vi "Rx Message to Transfer Handle - RT.vi"(8 "error in":errorcluster, 9 "message":T2={"name"="", "message type"="BC to RT", "endpoint Tx"={"terminal address"=0, "subaddress"=0}, "endpoint Rx"={"terminal address"=0, "subaddress"=0}, "create timestamp channel"=FALSE, "mode code"=0, "number of words"=0, "parameters"=[]}, 11 "remote terminal handles":u64[](array[numeric])) -> (0 "error out":errorcluster, 2 "valid?":bool, 3 "Rx read info":T1)   [LabVIEW 2020, in "AIM MIL-STD-1553 Engine.lvlib" / "Implementation.lvlib" / "Rx Execution Unit.lvclass"]
uses:
  Rx Execution Unit.lvclass
  <instrlib>/BTI1553Lib/BTI1553LV.lvlib
  <instrlib>/BTI1553Lib/Public/Controls/1553 RT Transfer Type.ctl
  <instrlib>/BTI1553Lib/Public/Controls/1553 Transfer Direction.ctl
  Shared/Rx Read Info.ctl
  <instrlib>/BTI1553Lib/Private/RT/Configure/Get RT Xfer Handle.vi
  Shared/Address.ctl
  Shared/Terminal Endpoint.ctl
  Shared/Parameter Definition.ctl
  Shared/Message Type.ctl
  Shared/Message Definition.ctl
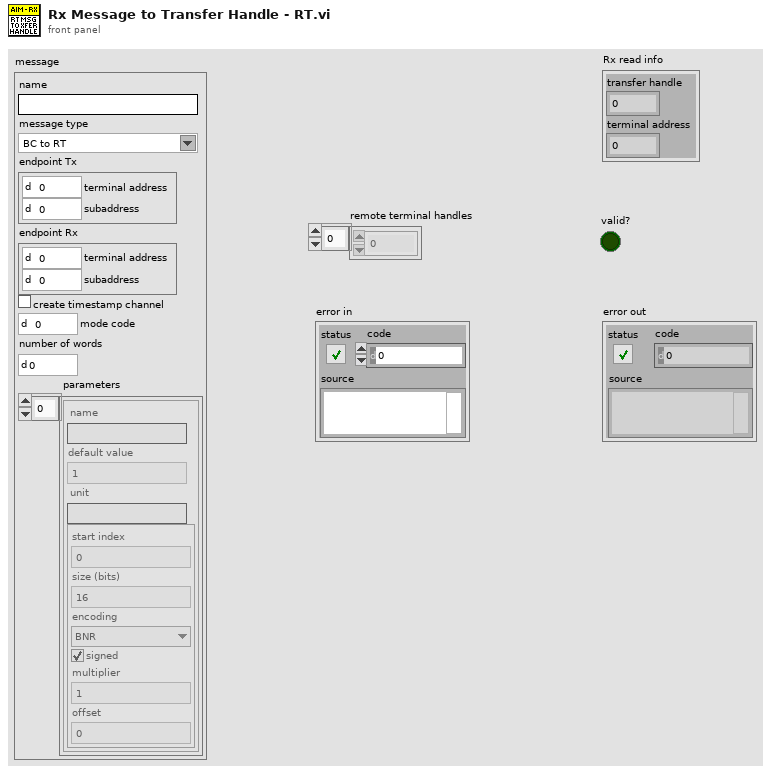
[diagram p1: front panel]
types:
  T1 = typedef "Rx Read Info.ctl" = cluster{"transfer handle":u64, "terminal address":u16}
  T2 = typedef "Message Definition.ctl" = cluster{"name":string, "message type":T3, "endpoint Tx":T4, "endpoint Rx":T4, "create timestamp channel":bool, "mode code":u16, "number of words":u16, "parameters":cluster{"name":string, "default value":dbl, "unit":string, "parameter definition":T6}[]}
  T3 = typedef "Message Type.ctl" = string
  T4 = typedef "Terminal Endpoint.ctl" = cluster{"terminal address":T5, "subaddress":T5}
  T5 = typedef "Address.ctl" = u16
  T6 = typedef "Parameter Definition.ctl" = cluster{"start index":i32, "size (bits)":i32, "encoding":enum16{"BNR", "BCD", "Discrete"}, "signed":bool, "multiplier":dbl, "offset":dbl}
  T7 = typedef "BTI1553LV.lvlib/1553 RT Transfer Type.ctl" = u32
  T8 = typedef "BTI1553LV.lvlib/1553 Transfer Direction.ctl" = u32
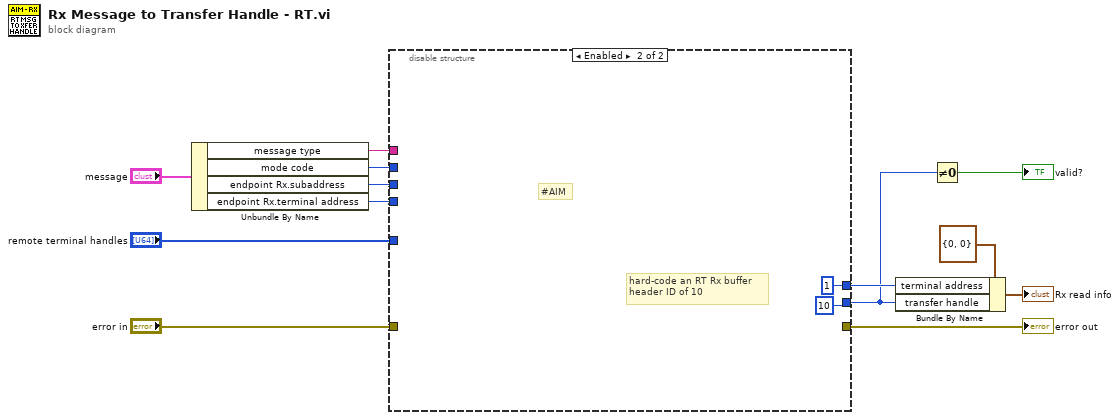
[diagram p0: block diagram]
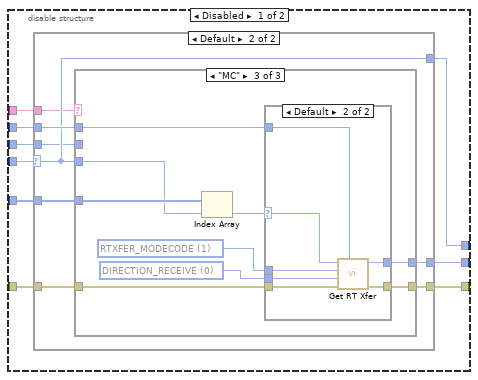
[diagram p2: hidden frame]
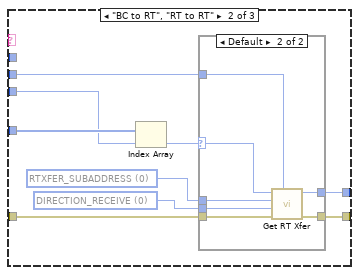
[diagram p5: hidden frame]
diagram:
  n1 = Unbundle By Name("message") -> ("message type"=w2:T3, "mode code"=w11:u16, "endpoint Rx.subaddress"=w1:T5, "endpoint Rx.terminal address"=w13:T5)
  n2 = disable-structure shown="Enabled" {
    disable-tunnel: w13 -> [w22 _]
    disable-tunnel: w11 -> [w21 _]
    disable-tunnel: "error in" -> [w20 _]
    disable-tunnel: "remote terminal handles" -> [w19 _]
    disable-tunnel: [w18 _] -> w8
    disable-tunnel: [w17 T5 1 ("terminal address")] -> w5
    disable-tunnel: [w16 u64 10 ("rt transfer handle out")] -> w3
    disable-tunnel: w2 -> [w15 _]
    disable-tunnel: w1 -> [w14 _]
    frame Disabled {
      n3 = case shown="Default" w22 {
        selector: w22 -> [_ w26]
        tunnel: w20 -> [w23 w31]
        tunnel: [w23 w30] -> w18
        tunnel: w19 -> [_ w29]
        tunnel: w21 -> [_ w28]
        tunnel: [_ w27] -> w16
        tunnel: [_ w26] -> w17
        tunnel: w15 -> [_ w25]
        tunnel: w14 -> [_ w24]
        frame 0 {
        }
        frame Default {
          n4 = case shown="\"MC\"" w25 {
            tunnel: w31 -> [w32 w41 w58]
            tunnel: [w32 w40 w57] -> w30
            tunnel: w29 -> [_ w37 w54]
            tunnel: w28 -> [_ _ w52]
            tunnel: [_ w35 w51] -> w27
            tunnel: w26 -> [_ w34 w50]
            tunnel: w24 -> [_ w33 _]
            frame Default {
            }
            frame "BC to RT", "RT to RT" {
              w38 = T7 0 items=["RTXFER_SUBADDRESS", "RTXFER_MODECODE"] ("transfer type")
              w39 = T8 0 items=["DIRECTION_RECEIVE", "DIRECTION_TRANSMIT"] ("transfer direction")
              n5 = Index Array(array=w37, index=w34) -> (element=w36:u64)
              n6 = case shown="Default" w36 {
                selector: w36 -> [_ w45]
                tunnel: w41 -> [w42 w49]
                tunnel: [w42 w48] -> w40
                tunnel: w39 -> [_ w47]
                tunnel: w38 -> [_ w46]
                tunnel: [_ w44] -> w35
                tunnel: w33 -> [_ w43]
                frame 0, -1 {
                }
                frame Default {
                  n7 = call-poly <instrlib>:"Get RT Xfer.vi"("transfer sa number or mc number"=w43, "error in (no error)"=w49, "transfer direction"=w47, "transfer type"=w46, "remote terminal handle in"=w45) -> ("error out"=w48:errorcluster, "rt transfer handle out"=w44:u64)  [unwired: 4 in, 1 out]
                }
              }
            }
            frame "MC" {
              w55 = T7 1 items=["RTXFER_SUBADDRESS", "RTXFER_MODECODE"] ("transfer type")
              w56 = T8 0 items=["DIRECTION_RECEIVE", "DIRECTION_TRANSMIT"] ("transfer direction")
              n8 = Index Array(array=w54, index=w50) -> (element=w53:u64)
              n9 = case shown="Default" w53 {
                selector: w53 -> [_ w62]
                tunnel: w58 -> [w59 w66]
                tunnel: [w59 w65] -> w57
                tunnel: w56 -> [_ w64]
                tunnel: w55 -> [_ w63]
                tunnel: w52 -> [_ w61]
                tunnel: [_ w60] -> w51
                frame 0, -1 {
                }
                frame Default {
                  n10 = call-poly <instrlib>:"Get RT Xfer.vi"("transfer sa number or mc number"=w61, "error in (no error)"=w66, "transfer direction"=w64, "transfer type"=w63, "remote terminal handle in"=w62) -> ("error out"=w65:errorcluster, "rt transfer handle out"=w60:u64)  [unwired: 4 in, 1 out]
                }
              }
            }
          }
        }
      }
    }
    frame Enabled {
      # "#AIM"
      # "hard-code an RT Rx buffer\nheader ID of 10"
    }
  }
  "error out" <- w8
  n11 = Bundle By Name(cluster=T1 {"transfer handle"=0, "terminal address"=0} ("Rx read info"), "terminal address"=w5, "transfer handle"=w3) -> (→"Rx read info":T1)
  n12 = Not Equal To 0?(x=w3) -> (x != 0?=→"valid?":bool)
